vi "Koheras_AOTF-Init.vi"(11 "Koheras-AOTF-Controller":refnum<visa-resource-name>) -> (0 "error out":errorcluster, 3 "read buffer":string)   [LabVIEW 2009]
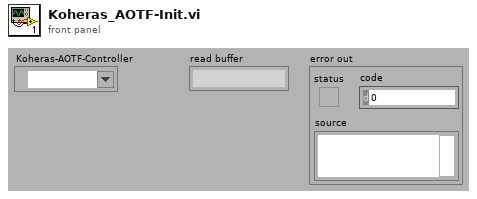
[diagram p1: front panel]
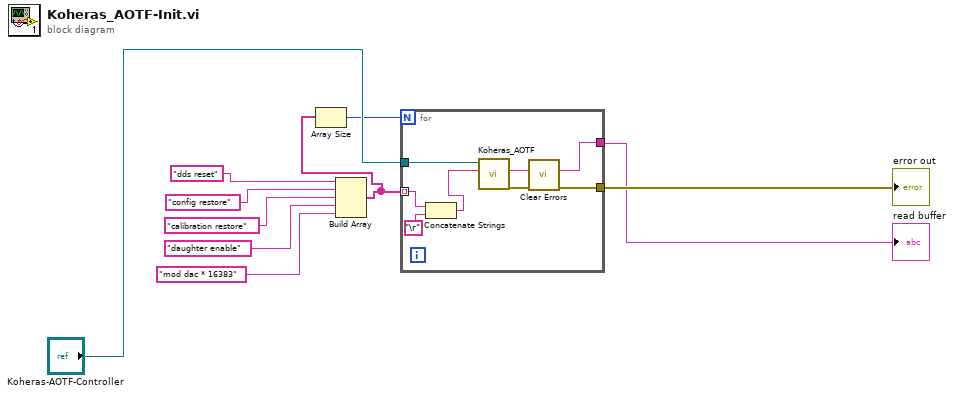
[diagram p0: block diagram]
diagram:
  n1 = Build Array("dds reset" ("string"), "config restore" ("string"), "calibration restore" ("string"), "daughter enable" ("string"), "mod dac * 16383" ("string")) -> (w2:string[])
  n2 = Array Size(array=w2) -> (size(s)=w1:i32)
  n3 = for {
    N: w1 -> [_]
    tunnel: [w17] -> w10
    tunnel: "Koheras-AOTF-Controller" -> [w16]
    tunnel: [w15] -> w8
    tunnel: w2 -> [w13] mode=indexing
    n4 = Concatenate Strings(w13, "\r") -> (w12:string)
    n5 = call "Koheras_AOTF.vi"("String"=w12, "VISA resource name 2"=w16) -> ("error out"=w14:errorcluster, "read buffer"=w15:string)  [unwired: 8 out]
    n6 = call <vilib>:"Clear Errors.vi"("error in (no error)"=w14) -> ("error out"=w17:errorcluster)  [unwired: 6 out]
  }
  "error out" <- w10
  "read buffer" <- w8
